vi "test Statically-sized Cluster Array Type.vi"(8 "error in (no error)":errorcluster, 11 "TestCase in":refnum<class "Malleable Tests.lvclass">) -> (0 "error out":errorcluster, 3 "TestCase out":refnum<class "Malleable Tests.lvclass">)   [LabVIEW 2020, in "Memory Manager Tests.lvlib" / "Malleable Tests.lvclass"]
uses:
  Malleable Tests.lvclass
  <vilib>/addons/_JKI Toolkits/VI Tester/TestCase.llb/TestCase.lvclass
  Malleable Type Tests/Statically-sized Cluster Array.vi
  Malleable Type Tests/Malleable Type Tests.lvclass
  C:/Program Files (x86)/National Instruments/LabVIEW 2020/vi.lib/addons/_JKI Toolkits/VI Tester/TestCase.llb/TestCase.lvclass
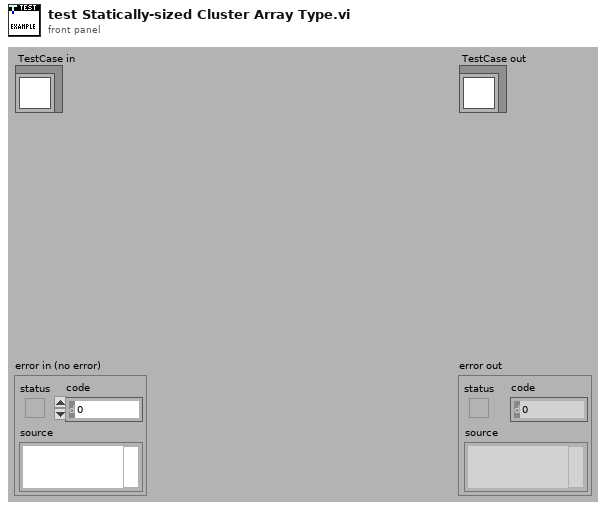
[diagram p1: front panel]
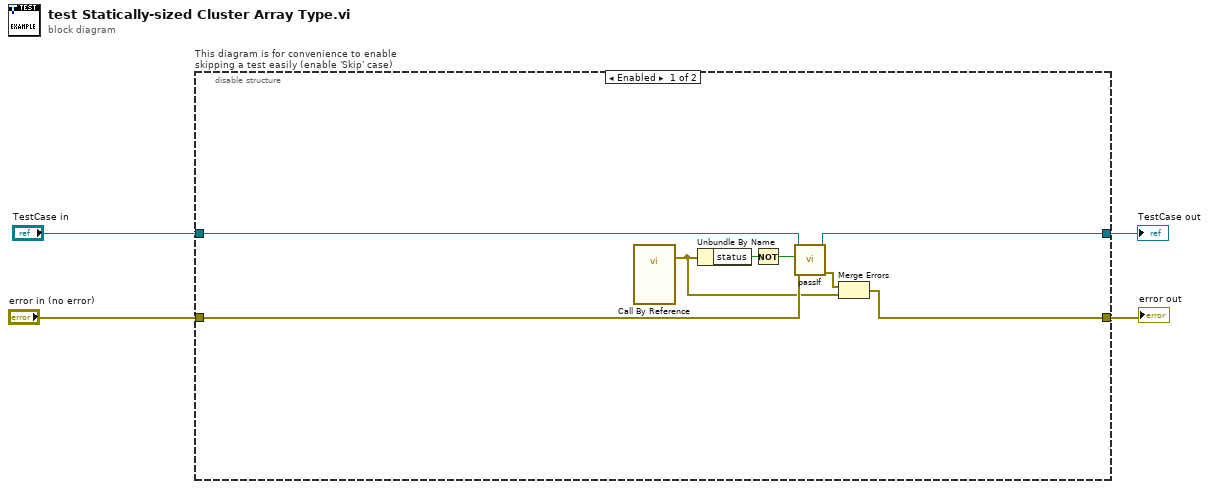
[diagram p0: block diagram]
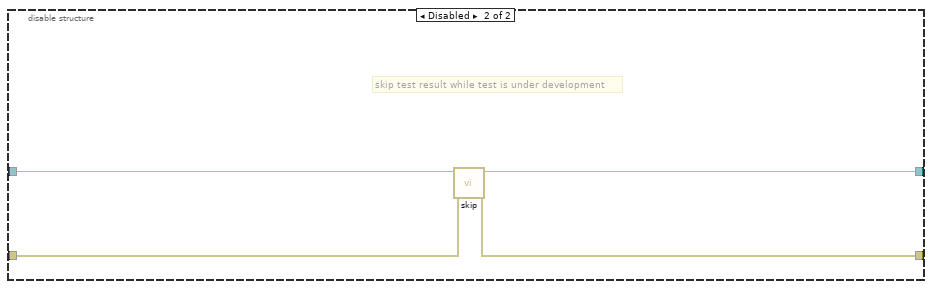
[diagram p2: hidden frame]
diagram:
  n1 = disable-structure "This diagram is for convenience to enable skipping a test easily (enable 'Skip' case)" shown="Enabled" {
    disable-tunnel: "TestCase in" -> [w12 w16]
    disable-tunnel: [w11 w14] -> w1
    disable-tunnel: [w6 w15] -> w3
    disable-tunnel: "error in (no error)" -> [w7 w13]
    frame Enabled {
      n2 = call-by-ref "?"() -> (error out=w5:errorcluster)  [unwired: 14 in, 1 out]
      n3 = Unbundle By Name(w5) -> ("status"=w9:bool)
      n4 = Not(x=w9) -> (.not. x?=w8:bool)
      n5 = call-dynamic "passIf.vi"("error in (no error)"=w7, "pass"=w8, "TestCase in"=w12) -> ("error out"=w10:errorcluster, "TestCase out"=w11:refnum<class "Malleable Tests.lvclass">)  [unwired: 7 in]
      n6 = Merge Errors(w10, w5) -> (w6:errorcluster)
    }
    frame Disabled {
      # "skip test result while test is under development"
      n7 = call <vilib>:"skip.vi"("error in (no error)"=w13, "TestCase in"=w16) -> ("error out"=w15:errorcluster, "TestCase out"=w14:refnum<class "Malleable Tests.lvclass">)  [unwired: 8 in]
    }
  }
  "error out" <- w3
  "TestCase out" <- w1
